vi "Fuel Injector Measurement Type Section.vi"(8 "error in (no error)":errorcluster, 11 "Node Ptr":T1 format="%.0x") -> (0 "error out":errorcluster)   [LabVIEW 2019, in "Fuel Injector Analysis Addon System Explorer.lvlib"]
uses:
  Fuel Injector Analysis Addon System Explorer.lvlib
  <vilib>/NI VeriStand/Custom Device API/Custom Device Item Ref.ctl
  Addon Shared/Constants.vi
  <vilib>/NI VeriStand/Custom Device Tools/Custom Device Utility Library/NI VeriStand - Search for All Items by GUID.vi
  <vilib>/NI VeriStand/Custom Device Tools/Custom Device Utility Library/NI VeriStand - Search for Item by GUID.vi
  <vilib>/NI VeriStand/Custom Device API/Custom Device API.lvlib
  <vilib>/NI VeriStand/Custom Device Tools/Custom Device Utility Library/Custom Device Utility Library.lvlib
  Addon Shared/Fuel Injector Analysis Addon Shared.lvlib
panel:
  in  "Sample Rate (Hz)":u32
  out "Original Name":string
  out "Available Registers":i32[](listbox)
  in  "Settings":bool
  in  "SHDocVw.IWebBrowser":refnum<k7>(container)
  in  "Header":cluster{"Section Name":string}={"Section Name"="Custom Device Item Settings"}
  in  "Description":string
  in  "Name":string
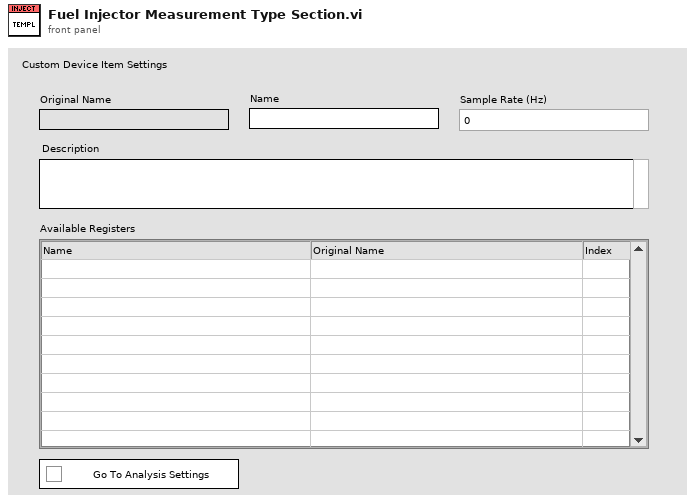
[diagram p1: front panel]
types:
  T1 = typedef "Custom Device API.lvlib/Custom Device Item Ref.ctl" = u64
  T2 = typedef "Custom Device API.lvlib/Custom Device Item Info.ctl" = cluster{"Name":string, "Is Channel":bool, "GUID":string, "Is Waveform":bool}
  T3 = typedef "Custom Device API.lvlib/Custom Device Commands.ctl" = enum16{"Default", "Item renamed", "Shutdown", "Dynamic button pressed"}
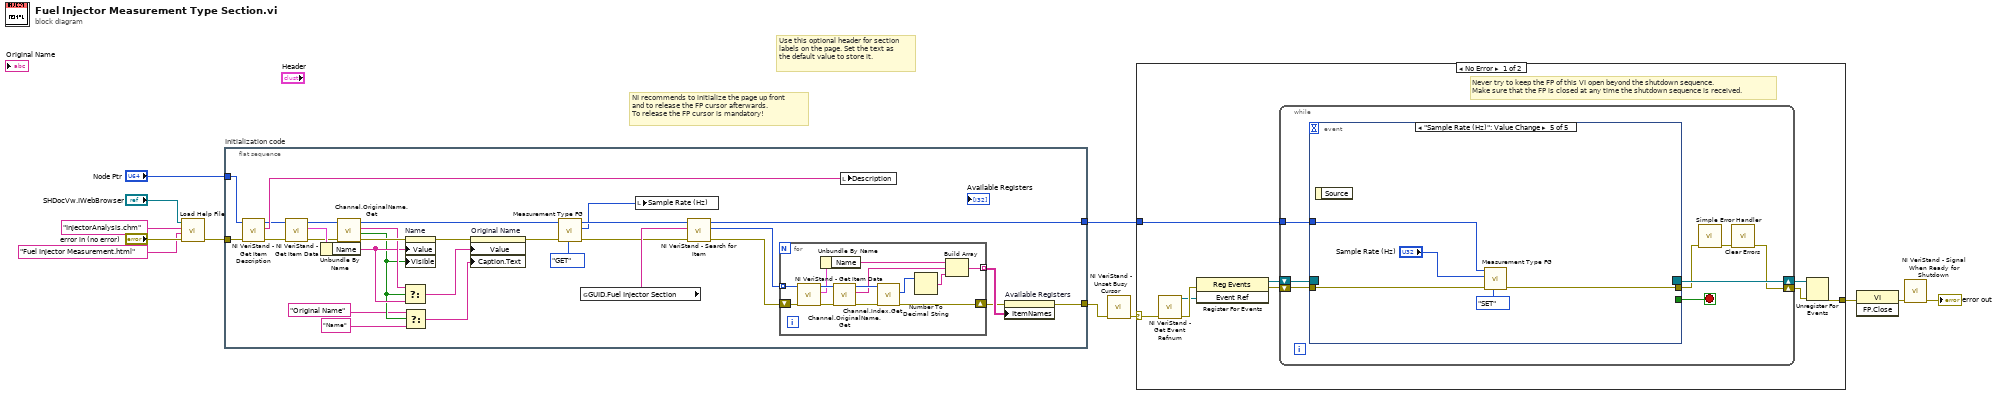
[diagram p0: block diagram]
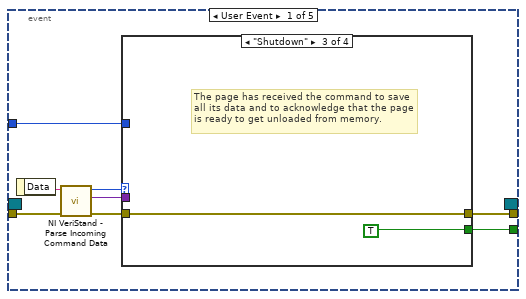
[diagram p2: hidden frame]
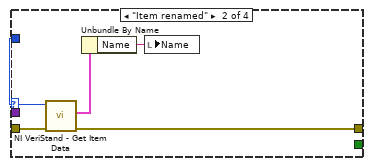
[diagram p4: hidden frame]
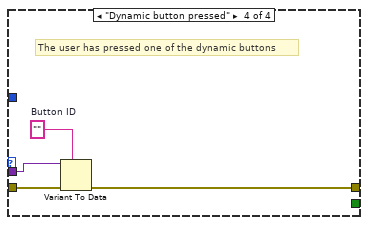
[diagram p5: hidden frame]
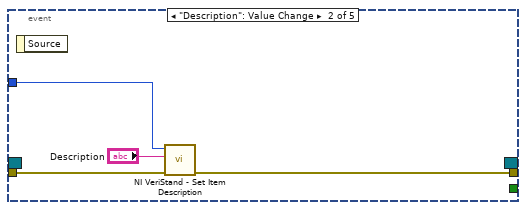
[diagram p6: hidden frame]
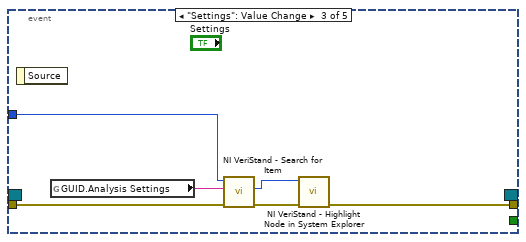
[diagram p7: hidden frame]
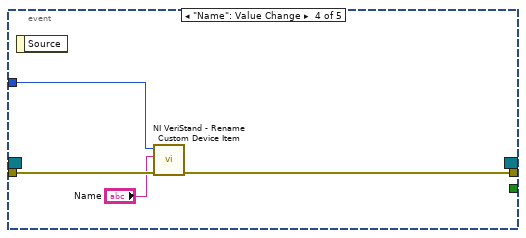
[diagram p8: hidden frame]
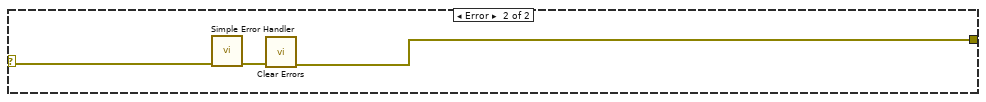
[diagram p9: hidden frame]
diagram:
  # "Use this optional header for section labels on the page. Set the text as the default value to store it."
  # "NI recommends to initialize the page up front\nand to release the FP cursor afterwards.\nTo release the FP cursor is mandatory!"
  n1 = call "Load Help File.vi"("error in (no error)"="error in (no error)", "HTML File"="Fuel Injector Measurement.html" ("Main CHM File"), "Main CHM File"="InjectorAnalysis.chm", "SHDocVw.IWebBrowser2"="SHDocVw.IWebBrowser") -> ("error out"=w4:errorcluster)  [unwired: 7 in]
  n2 = flat-sequence "Initialization code" {
    tunnel: w4 -> [w42]
    tunnel: [w34] -> w9
    tunnel: [w39] -> w7
    tunnel: "Node Ptr" -> [w40]
    frame #0 {
      n3 = call <vilib>:"NI VeriStand - Get Item Description.vi"("error in (no error)"=w42, "Item Ref in"=w40) -> ("error out"=w21:errorcluster, "Description"=w41:string, "Item Ref out"=w20:T1)  [unwired: 7 out]
      n4 = call <vilib>:"NI VeriStand - Get Item Data.vi"("error in (no error)"=w21, "Item Ref in"=w20) -> ("error out"=w31:errorcluster, "Item Info"=w33:T2, "Item Ref out"=w32:T1)  [unwired: 7 out]
      n5 = Unbundle By Name(w33) -> ("Name"=w27:string)
      n6 = call "Channel.OriginalName.Get.vi"("error in (no error)"=w31, "Ref in"=w32) -> ("error out"=w30:errorcluster, "Found?"=w25:bool, "Value"=w28:string, "Ref out"=w17:T1)  [unwired: 6 in]
      n7 = Select(t=w28, s=w25, f=w27) -> (s? t:f=w26:string)
      n8 = Select(t="Original Name" ("s? t:f"), s=w25, f="Name" ("s? t:f")) -> (s? t:f=w22:string)
      n9 = property on="Name" class="Str"(error in=w30, "Value"=w27, "Visible"=w25) -> (error out=w29:errorcluster)  [unwired: 1 in, 1 out]
      n10 = property on="Original Name" class="Str"(error in=w29, "Value"=w26, "Caption.Text"=w22) -> (error out=w18:errorcluster)  [unwired: 1 in, 1 out]
      n11 = call "Measurement Type FG.vi"("Action"=enum8{"GET", "SET"}."GET", "error in (no error)"=w18, "Item Ref"=w17) -> ("error out"=w15:errorcluster, "Sample rate (S/s)"=w13:u32, "Item Ref out"=w16:T1)  [unwired: 6 in]
      n12 = global read "Constants.vi" "GUID.Fuel Injector Section"() -> (w19:string)
      n13 = local write "Sample Rate (Hz)"(w13) -> ()
      n14 = call-poly <vilib>:"NI VeriStand - Search for Item.vi"("error in"=w15, "Item GUID"=w19, "Section Ref in"=w16) -> ("error out"=w37:errorcluster, "Item Refs"=w38:T1[], "Section Ref out"=w39:T1)  [unwired: 5 in, 1 out]
      n15 = for {
        tunnel: w38 -> [w55] mode=indexing
        shift-right: [w49] -> w35
        shift-left: w37 -> [w52]
        tunnel: [w43] -> w36 mode=indexing
        n16 = call <vilib>:"NI VeriStand - Get Item Data.vi"("error in (no error)"=w52, "Item Ref in"=w55) -> ("error out"=w51:errorcluster, "Item Info"=w48:T2, "Item Ref out"=w54:T1)  [unwired: 7 out]
        n17 = Unbundle By Name(w48) -> ("Name"=w47:string)
        n18 = call "Channel.OriginalName.Get.vi"("error in (no error)"=w51, "Ref in"=w54) -> ("error out"=w50:errorcluster, "Value"=w46:string, "Ref out"=w53:T1)  [unwired: 6 in, 1 out]
        n19 = call "Channel.Index.Get.vi"("error in (no error)"=w50, "Ref in"=w53) -> ("error out"=w49:errorcluster, "Value"=w45:u16)  [unwired: 6 in, 2 out]
        n20 = Number To Decimal String(number=w45) -> (decimal integer string=w44:string)  [unwired: 1 in]
        n21 = Build Array(w47, w46, w44) -> (w43:string[])
      }
      n22 = local write "Description"(w41) -> ()
      n23 = property on="Available Registers" class="MCListbox (strict)"(error in=w35, "ItemNames"=w36) -> (error out=w34:errorcluster)  [unwired: 1 in, 1 out]
    }
  }
  n24 = call <vilib>:"NI VeriStand - Unset Busy Cursor.vi"("error in (no error)"=w9) -> ("error out"=w8:errorcluster)  [unwired: 10 out]
  n25 = case shown="No Error" w8 {
    selector: w8 -> [w56 w114]
    tunnel: [w61 w112] -> w12
    tunnel: w7 -> [w57 _]
    frame No Error {
      # "Never try to keep the FP of this VI open beyond the shutdown sequence.\nMake sure that the FP is closed at any time the shutdown sequence is received."
      n26 = call <vilib>:"NI VeriStand - Get Event Refnum.vi"("error in (no error)"=w56) -> ("error out"=w64:errorcluster, "Event Ref"=w60:refnum<user-event>)  [unwired: 9 out]
      n27 = register-events(error in=w64, w60) -> (reference out=w58:refnum<event-registration>, error out=w59:errorcluster)  [unwired: 1 in]
      n28 = while {
        tunnel: w57 -> [w68]
        shift-right: [w65] -> w62
        shift-left: w59 -> [w71]
        shift-right: [w72] -> w63
        shift-left: w58 -> [w70]
        stop <- w69 stop-if-true
        n29 = event shown="[4] \"Sample Rate (Hz)\": Value Change" {
          selector: w70 -> [_ _ _ _ _]
          dyn-events: [_ _ _ _ _] -> w72
          timeout: _ -> [_ _ _ _ _]
          tunnel: w71 -> [w80 w95 w99 w105 w110]
          tunnel: [w76 _ _ _ _] -> w69
          tunnel: [w75 w94 w97 w104 w108] -> w67
          tunnel: w68 -> [w74 w96 w98 w106 w109]
          event User Event {
            n30 = event-data() -> ("Data"=w79:string)  [unwired: 1 out]
            n31 = call <vilib>:"NI VeriStand - Parse Incoming Command Data.vi"("error in (no error)"=w80, "Incoming data"=w79) -> ("error out"=w78:errorcluster, "Outgoing data"=w73:variant, "Action"=w77:T3)  [unwired: 7 out]
            n32 = case shown="\"Shutdown\"" w77 {
              tunnel: w78 -> [w81 w86 w87 w92]
              tunnel: [_ _ TRUE _] -> w76
              tunnel: [w81 w82 w87 w89] -> w75
              tunnel: w74 -> [_ w85 _ _]
              tunnel: w73 -> [_ _ _ w91]
              frame "Default", Default {
              }
              frame "Item renamed" {
                n33 = call <vilib>:"NI VeriStand - Get Item Data.vi"("error in (no error)"=w86, "Item Ref in"=w85) -> ("error out"=w82:errorcluster, "Item Info"=w84:T2)  [unwired: 8 out]
                n34 = Unbundle By Name(w84) -> ("Name"=w83:string)
                n35 = local write "Name"(w83) -> ()
              }
              frame "Shutdown" {
                # "The page has received the command to save all its data and to acknowledge that the page is ready to get unloaded from memory."
              }
              frame "Dynamic button pressed" {
                w90 = ""  # Button ID
                # "The user has pressed one of the dynamic buttons"
                n36 = Variant To Data(error in=w92, type=w90, Variant=w91) -> (error out=w89:errorcluster)  [unwired: 1 out]
              }
            }
          }
          event "Description": Value Change {
            n37 = event-data() -> ()  [unwired: 2 out]
            n38 = call <vilib>:"NI VeriStand - Set Item Description.vi"("error in (no error)"=w95, "Description"="Description", "Item Ref in"=w96) -> ("error out"=w94:errorcluster)  [unwired: 8 out]
          }
          event "Settings": Value Change {
            n39 = event-data() -> ()  [unwired: 2 out]
            n40 = global read "Constants.vi" "GUID.Analysis Settings"() -> (w102:string)
            n41 = call-poly <vilib>:"NI VeriStand - Search for Item.vi"("error in"=w99, "Item GUID"=w102, "Section Ref in"=w98) -> ("error out"=w101:errorcluster, "Item Ref"=w100:T1)  [unwired: 5 in, 2 out]
            n42 = call <vilib>:"NI VeriStand - Highlight Node in System Explorer.vi"("error in (no error)"=w101, "Item Ref in"=w100) -> ("error out"=w97:errorcluster)  [unwired: 8 in, 1 out]
          }
          event "Name": Value Change {
            n43 = event-data() -> ()  [unwired: 2 out]
            n44 = call <vilib>:"NI VeriStand - Rename Custom Device Item.vi"("error in (no error)"=w105, "New Name"="Name", "Item Ref in"=w106) -> ("error out"=w104:errorcluster)  [unwired: 6 in, 2 out]
          }
          event "Sample Rate (Hz)": Value Change {
            n45 = event-data() -> ()  [unwired: 2 out]
            n46 = call "Measurement Type FG.vi"("Action"=enum8{"GET", "SET"}."SET", "error in (no error)"=w110, "Sample rate (S/s)"="Sample Rate (Hz)", "Item Ref"=w109) -> ("error out"=w108:errorcluster)  [unwired: 5 in, 2 out]
          }
        }
        n47 = call <vilib>:"Simple Error Handler.vi"("error in (no error)"=w67) -> ("error out"=w66:errorcluster)  [unwired: 1 in, 7 out]
        n48 = call <vilib>:"Clear Errors.vi"("error in (no error)"=w66) -> ("error out"=w65:errorcluster)  [unwired: 1 in, 5 out]
      }
      n49 = Unregister For Events(event registration refnum=w63, error in=w62) -> (error out=w61:errorcluster)
    }
    frame Error {
      n50 = call <vilib>:"Simple Error Handler.vi"("error in (no error)"=w114) -> ("error out"=w113:errorcluster)  [unwired: 1 in, 7 out]
      n51 = call <vilib>:"Clear Errors.vi"("error in (no error)"=w113) -> ("error out"=w112:errorcluster)  [unwired: 1 in, 5 out]
    }
  }
  n52 = invoke class="VI" method="FP.Close"(error in=w12) -> (error out=w11:errorcluster)  [unwired: 2 in, 2 out]
  n53 = call <vilib>:"NI VeriStand - Signal When Ready for Shutdown.vi"("error in (no error)"=w11) -> ("error out"=→"error out":errorcluster)  [unwired: 10 out]
